vi "UpdateViCtrl.vi"(8 "error in (no error)":errorcluster, 10 "Controls":path, 11 "VIToUpdate":path) -> (0 "error out":errorcluster, 3 "reference out":refnum<vi>)   [LabVIEW 2018]
doc: "Update the controls in single vi."
uses:
  <vilib>/Utility/traverseref.llb/TRef TravTarget.ctl
  <vilib>/Utility/traverseref.llb/VI Scripting - Traverse.lvlib
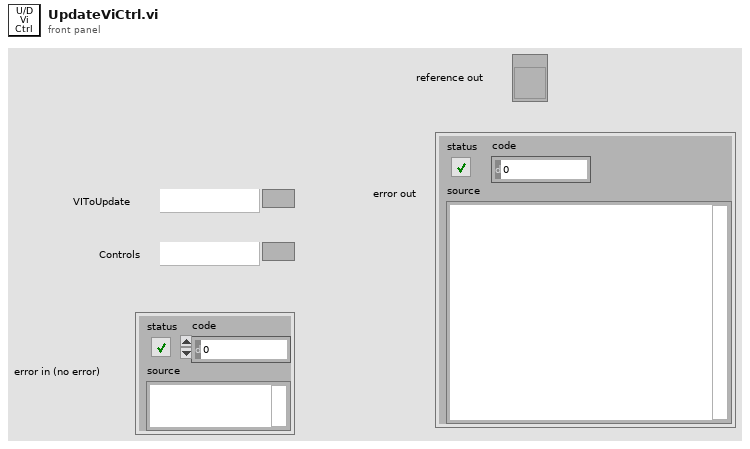
[diagram p1: front panel]
types:
  T1 = typedef "TRef TravTarget.ctl" = enum16{"FP", "BD", "Other"}
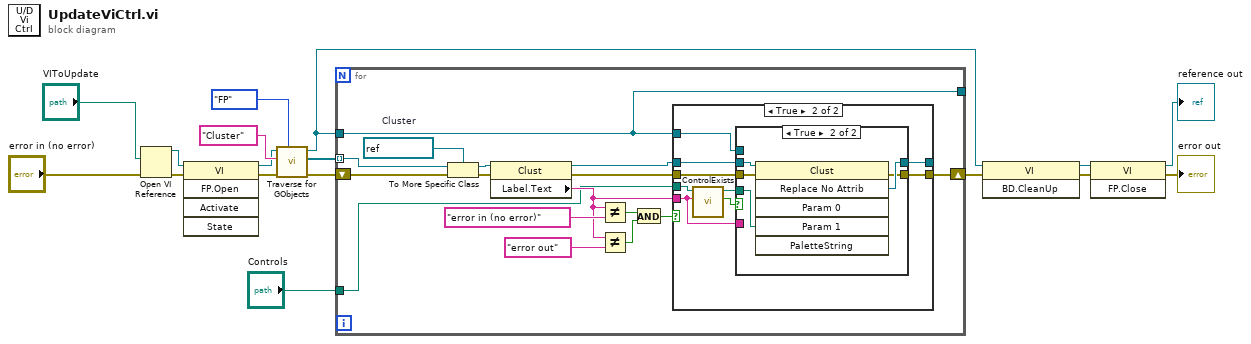
[diagram p0: block diagram]
diagram:
  n1 = Open VI Reference(vi path="VIToUpdate", error in (no error)="error in (no error)") -> (vi reference=w13:refnum<vi>, error out=w9:errorcluster)  [unwired: 4 in]
  n2 = invoke class="VI" method="FP.Open"(reference=w13, error in=w9) -> (reference out=w10:refnum<vi>, error out=w8:errorcluster)  [unwired: 3 in, 3 out]
  n3 = call <vilib>:"Traverse for GObjects.vi"("Traverse Target"=TRef_TravTarget."FP", "error in (no error)"=w8, "Class Name"="Cluster", "VI Refnum"=w10) -> ("error out"=w14:errorcluster, "References"=w15:refnum<vi>[], "dup VI Refnum"=w2:refnum<vi>)  [unwired: 4 in, 1 out]
  n4 = for {
    tunnel: w15 -> [w31] mode=indexing
    tunnel: w2 -> [w19]
    shift-right: [w18] -> w4
    shift-left: w14 -> [w32]
    tunnel: "Controls" -> [w20]
    tunnel: [w19] -> _
    w33 = refnum<vi> refnum  # Cluster
    n5 = To More Specific Class(target class=w33, reference=w31, error in=w32) -> (specific class reference=w30:refnum<vi>, error out=w29:errorcluster)
    n6 = property class="Clust"(reference=w30, error in=w29) -> (reference out=w21:refnum<vi>, error out=w23:errorcluster, "Label.Text"=w22:string)
    n7 = Not Equal?(x=w22, y="error in (no error)") -> (x != y?=w27:bool)
    n8 = Not Equal?(x=w22, y="error out") -> (x != y?=w28:bool)
    n9 = And(x=w27, y=w28) -> (x .and. y?=w24:bool)
    n10 = case shown="True" w24 {
      tunnel: w23 -> [w34 w44]
      tunnel: w22 -> [_ w39]
      tunnel: w21 -> [w35 w43]
      tunnel: [w34 w42] -> w18
      tunnel: [w35 w41] -> _
      tunnel: w20 -> [_ w40]
      tunnel: w19 -> [_ w36]
      frame False {
      }
      frame True {
        n11 = call "ControlExists.vi"("ControlName"=w39, "ControlsPath"=w40) -> ("Boolean"=w38:bool, "ControlPath"=w37:path)  [unwired: 8 in]
        n12 = case shown="True" w38 {
          tunnel: w44 -> [w46 w49]
          tunnel: w43 -> [w45 w50]
          tunnel: [w46 w47] -> w42
          tunnel: [w45 w48] -> w41
          tunnel: w39 -> [_ _]
          tunnel: w37 -> [_ w51]
          tunnel: w36 -> [_ _]
          frame False {
          }
          frame True {
            n13 = invoke class="Clust" method="Replace No Attrib"(reference=w50, error in=w49, "Param 1"=w51) -> (error out=w47:errorcluster, "RepNoAttrib"=w48:refnum<vi>)  [unwired: 3 in, 4 out]
          }
        }
      }
    }
  }
  n14 = invoke class="VI" method="BD.CleanUp"(reference=w2, error in=w4) -> (reference out=w12:refnum<vi>, error out=w11:errorcluster)  [unwired: 1 in, 1 out]
  n15 = invoke class="VI" method="FP.Close"(reference=w12, error in=w11) -> (reference out=→"reference out":refnum<vi>, error out=→"error out":errorcluster)  [unwired: 1 in, 1 out]
